vi "PhotonCamera_GetDistCoeffs.vi"(11 "CameraName":string) -> (0 "error out":errorcluster, 3 "Dist Coeffs":T1)   [LabVIEW 2019, in "PhotonVisionLib.lvlib"]
doc: "Returns the distortion coeeficitions\n\nInputs:\n - cameraName -- The nickname of the camera (found in the PhotonVision UI).\n \nOutputs:\n - DistCoeffs - matrix - 5 x 1 matrix of distortion coefficients. If empty, nothing was returned or nothing exists."
uses:
  PhotonVisionLib.lvlib
  <vilib>/Analysis/Matrix/Datatypes/RealMatrix.ctl
  <vilib>/Rock Robotics/WPI/ThirdParty/JAS_Junk/TrajLib/MatBuilder_Create.vi
  <vilib>/Rock Robotics/Network Tables/NT Read Numeric Array.vi
  <vilib>/Rock Robotics/WPI/ThirdParty/JAS_Junk/TrajLib/Trajectory_Library.lvlib
  <vilib>/Analysis/Matrix/NI_Matrix.lvlib
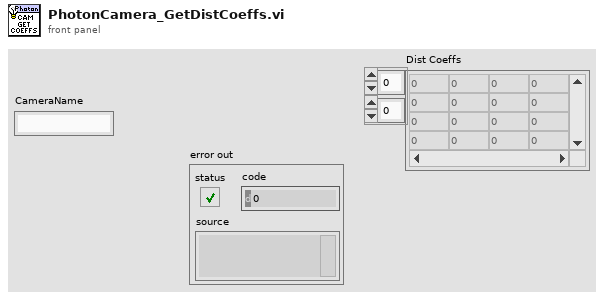
[diagram p1: front panel]
types:
  T1 = typedef "NI_Matrix.lvlib/RealMatrix.ctl" = dbl[][]
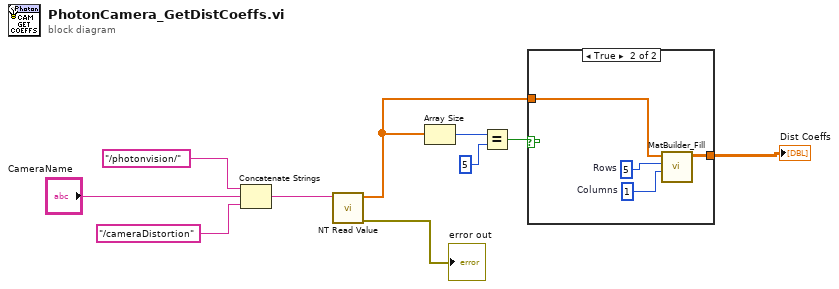
[diagram p0: block diagram]
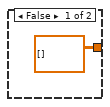
[diagram p2: hidden frame]
diagram:
  n1 = Concatenate Strings("/photonvision/", "CameraName", "/cameraDistortion") -> (w7:string)
  n2 = call-poly <vilib>:"NT Read Value.vi"("name"=w7) -> ("error out"=→"error out":errorcluster, "value"=w2:dbl[])  [unwired: 8 in, 1 out]
  n3 = Array Size(array=w2) -> (size(s)=w5:i32)
  n4 = Equal?(x=w5, y=5) -> (x = y?=w3:bool)
  n5 = case shown="True" w3 {
    tunnel: w2 -> [_ w13]
    tunnel: [T1 [] ("output matrix") w12] -> w1
    frame False {
    }
    frame True {
      w15 = 1  # Columns
      w14 = 5  # Rows
      n6 = call <vilib>:"MatBuilder_Fill.vi"("Columns"=w15, "Rows"=w14, "Value List"=w13) -> ("output matrix"=w12:T1)  [unwired: 8 in]
    }
  }
  "Dist Coeffs" <- w1
